vi "Event Log.vi"(11 "Module Config":T1={"Name"="Log", "Parent Q"=refnum, "Is Child?"=FALSE, "Index"=0, "Dirs"={"Root"=path "", "Config"=path "", "Logs"=path "", "Reports"=path "", "App Data"=path ""}, "Simulate"=FALSE, "SimCtrl"=refnum}) -> ()   [LabVIEW 2024, in "EQMF.lvlib" / "Event Log.lvlib"]
uses:
  Event Log.lvlib
  Module/Module Config.ctl
  Queues/Q.Element.ctl
  Module/Module.Working Dirs.ctl
  Module/Module.SW Version Info.ctl
  Module/Window/Window.Task, Action.ctl
  Event Log.Error Report.ctl
  Queues/Queue Utils.lvlib
  Module/Module Utils.lvlib
  Files/File Utils.lvlib
  Controls/Controls.lvlib
panel:
  in  "Main Tab":enum32{"Operate", "Maint"}(tab)
  in  "Clear Errors":bool
  out "Error Count":i32
  out "Log File":path
  in  "Auto Scroll":bool
  out "Event Log":string
  in  "Open Log Folder":bool
  in  "Clear":bool
  in  "Show Block Diagram":bool
  in  "Leave Maint":bool
  in  "Maint":bool
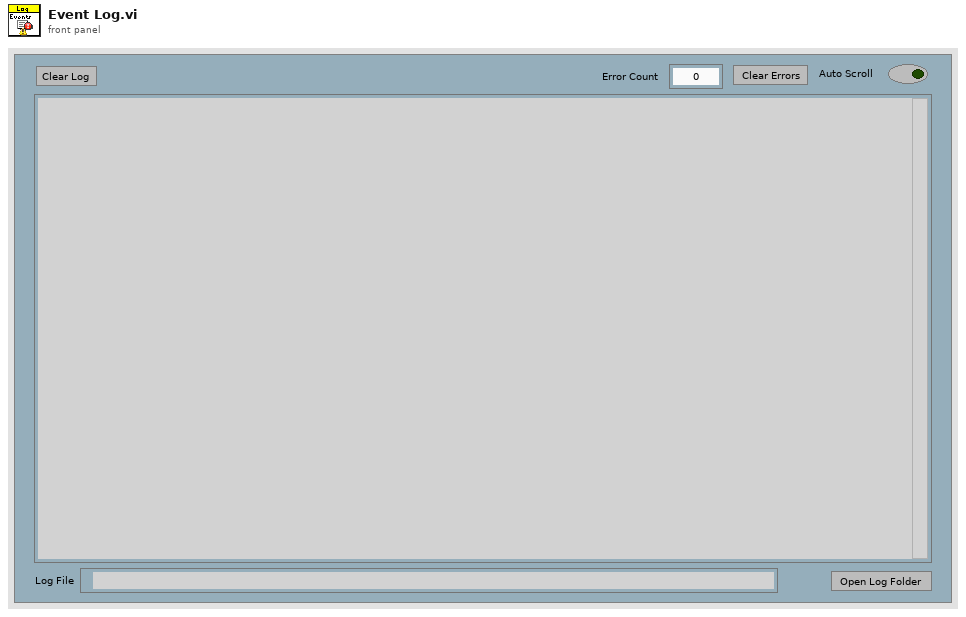
[diagram p1: front panel]
types:
  T1 = typedef "EQMF.lvlib/Module Utils.lvlib/Module Config.ctl" = cluster{"Name":string, "Parent Q":refnum<queue>, "Is Child?":bool, "Index":i32, "Dirs":T2, "Simulate":bool, "SimCtrl":refnum<vi>}
  T2 = typedef "EQMF.lvlib/Module Utils.lvlib/Module.Working Dirs.ctl" = cluster{"Root":path, "Config":path, "Logs":path, "Reports":path, "App Data":path}
  T3 = typedef "EQMF.lvlib/Module Utils.lvlib/Module.SW Version Info.ctl" = cluster{"AppName":string, "Company":string, "Version":string, "Description":string, "PN":string}
  T4 = typedef "EQMF.lvlib/Module Utils.lvlib/Module Sys Info.ctl" = cluster{"Main Q":refnum<queue>, "Exe":bool, "SW Rev":T3, "Self Ref":refnum<vi>, "Main Tab":refnum<vi>, "Pane":refnum<vi>, "Stop":cluster{"Ref":refnum<event-registration>, "Event":refnum<user-event>}, "Cfg":T1, "Services":cluster{"Name":string, "vi ref":refnum<vi>}[], "Menu Ref":refnum<k9>, "CtrlStates":refnum<class "Class.SaveCtrls.lvclass">, "Docs":cluster{"Tags":string[], "Paths":path[]}, "Log":refnum<class "Event Notification.lvclass">, "Test Controls":refnum<vi>[], "Child Modules":cluster{"Name":string, "vi ref":refnum<vi>}[], "SW Items":string[][], "AppData":refnum<class "Class.AppData.lvclass">, "Subscriptions":refnum<class "Subscription.lvclass">, "Module Config Ref":refnum<vi>}
  T5 = typedef "EQMF.lvlib/Module Utils.lvlib/Window.Task, Action.ctl" = enum16{"Resize()", "Show Panel(Bool)", "Show Scroll Bars(Bool)", "Dock to SubPanel(SubPanel Ref)", "Undock from SubPanel()", "Return to SubPanel()", "Go To Maint Tab()", "Show Maint Tab(Bool)", "Open Block Diagram()"}
  T6 = enum16{"Top Left", "Top Right", "Bottom Left", "Bottom Right"}
  T7 = enum16{"Top Left", "Top Right", "Bottom Left", "Bottom Right", "Left", "Right", "Top", "Bottom"}
  T8 = enum16{"open", "replace", "create", "open or create", "replace or create", "replace or create with confirmation"}
  T9 = cluster{"Log":string, "File Ref":refnum<file>, "File Date":string, "Parent Name":string}
  T10 = typedef "EQMF.lvlib/Event Log.lvlib/Event Log.Error Report.ctl" = cluster{"Cnt":i32, "Recent Error":errorcluster}
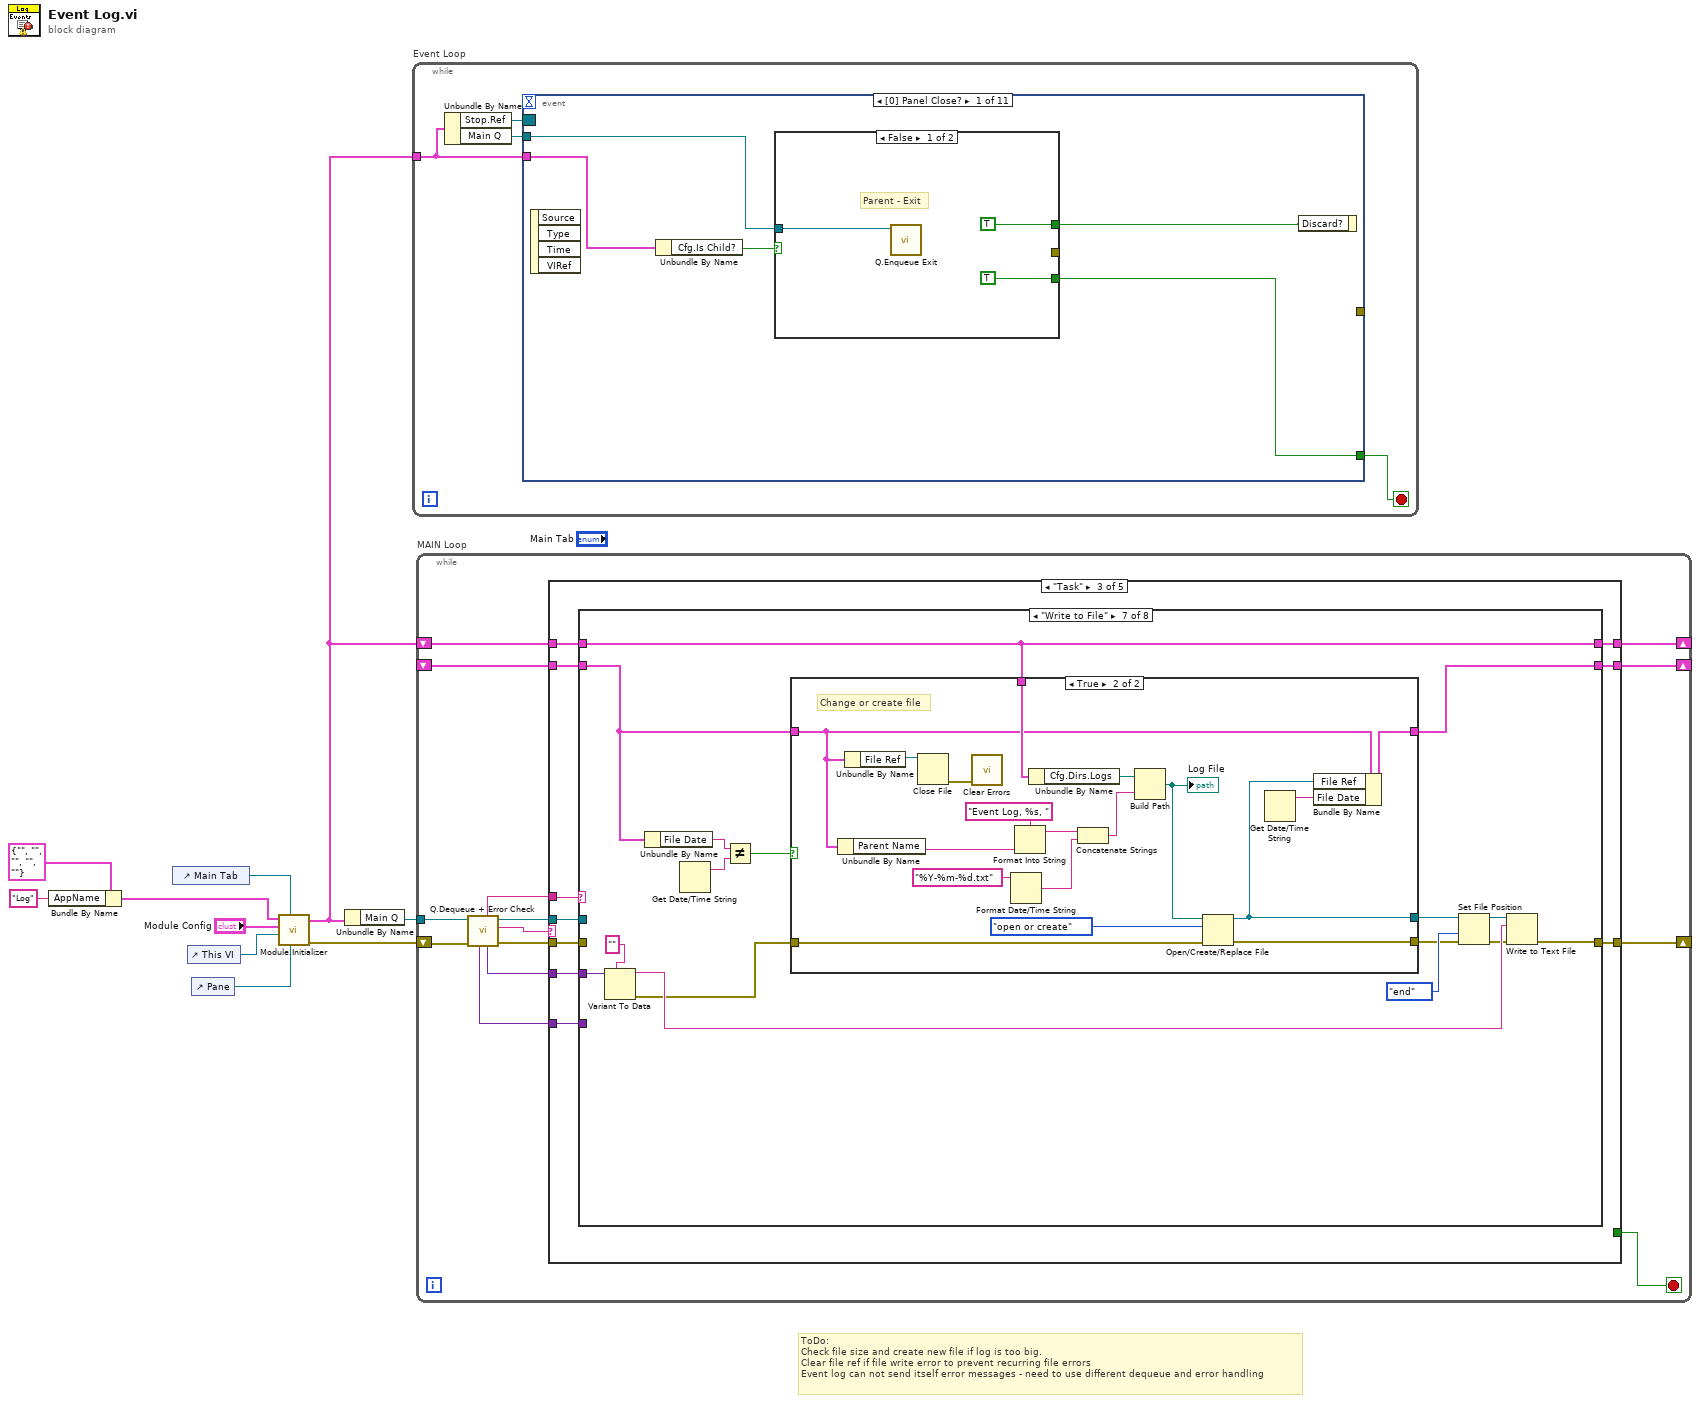
[diagram p0: block diagram]
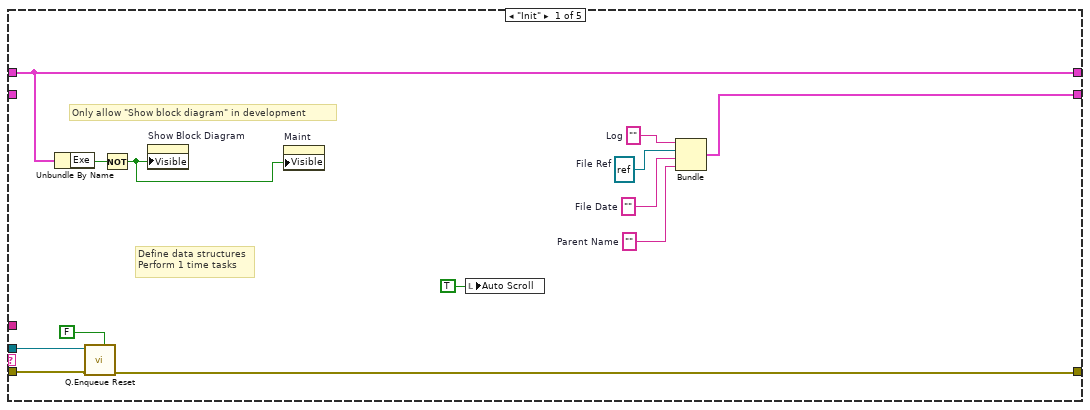
[diagram p2: hidden frame]
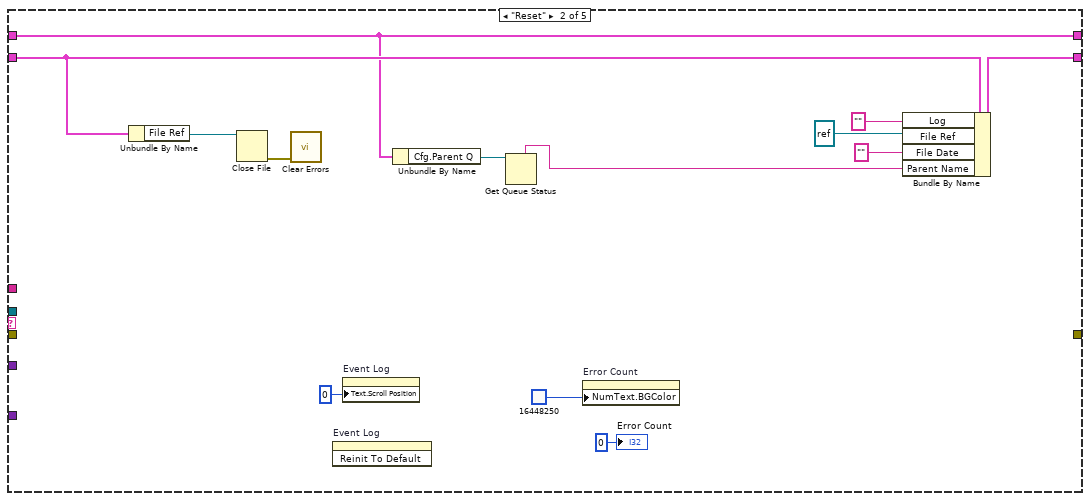
[diagram p3: hidden frame]
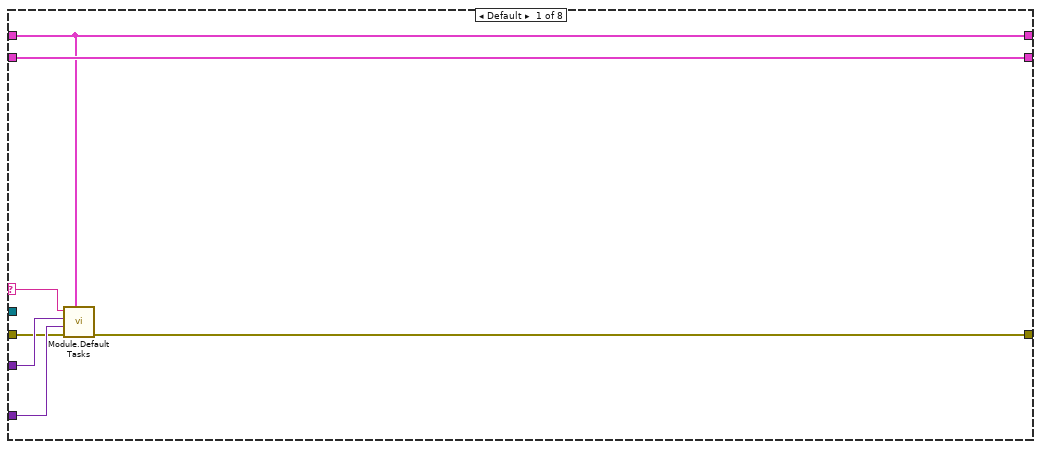
[diagram p4: hidden frame]
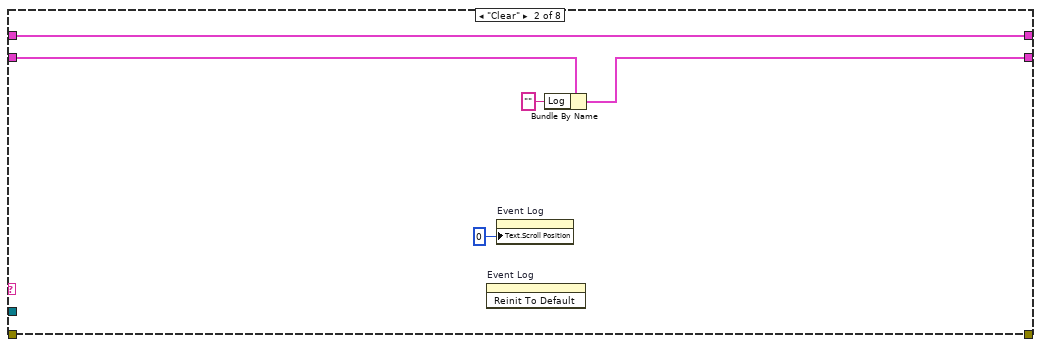
[diagram p5: hidden frame]
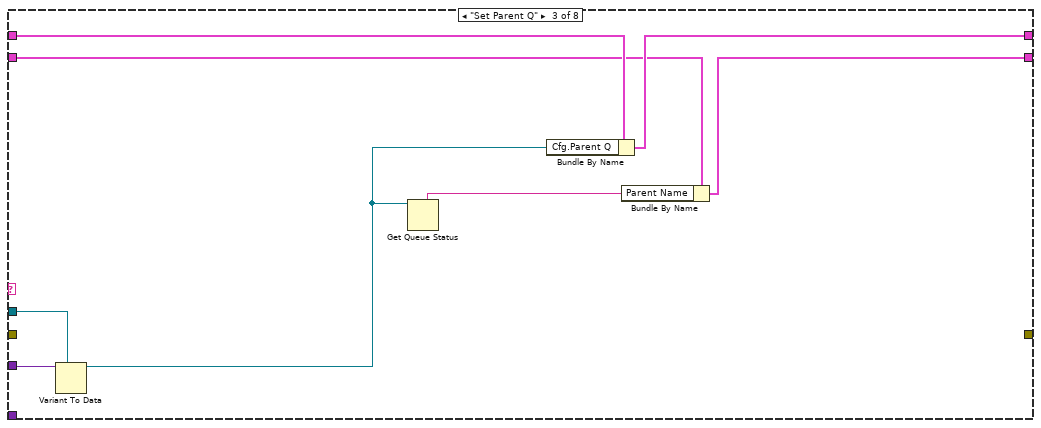
[diagram p6: hidden frame]
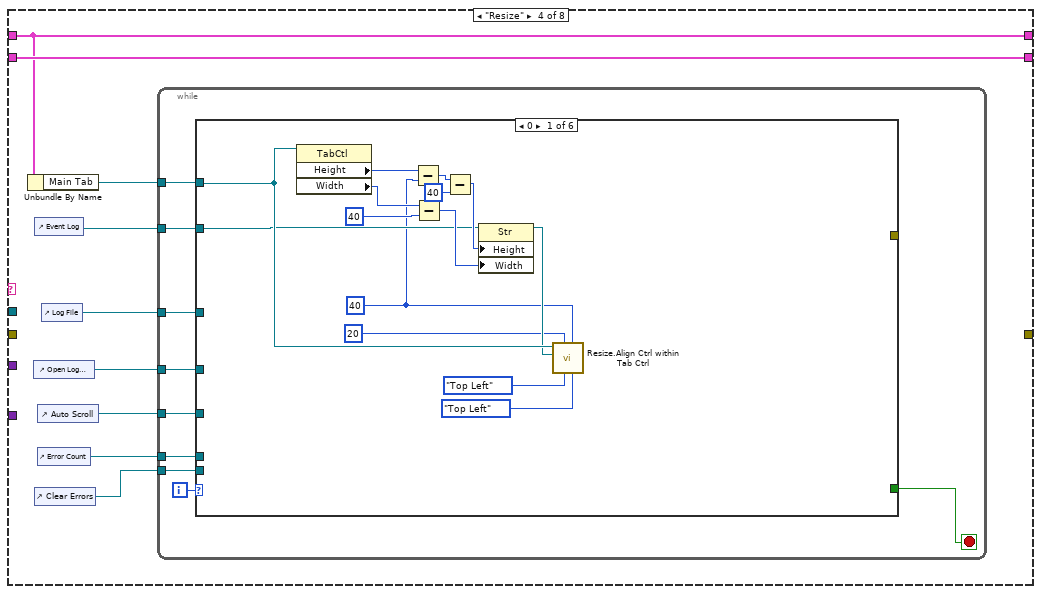
[diagram p7: hidden frame]
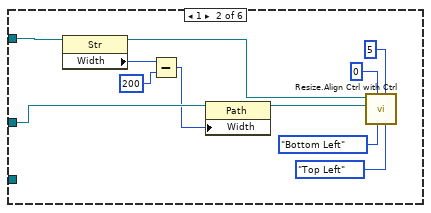
[diagram p8: hidden frame]
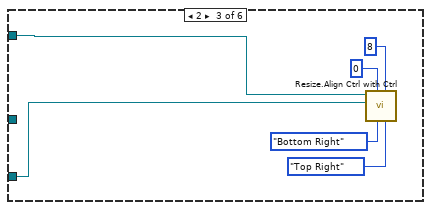
[diagram p9: hidden frame]
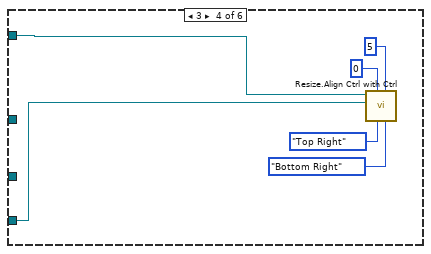
[diagram p10: hidden frame]
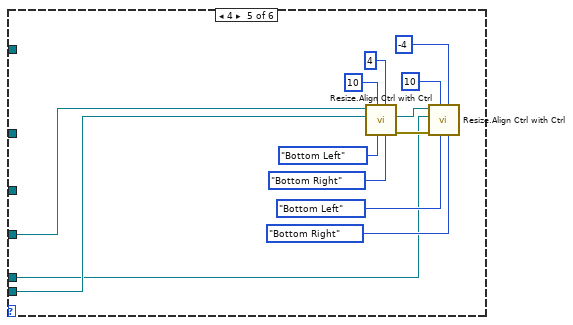
[diagram p11: hidden frame]
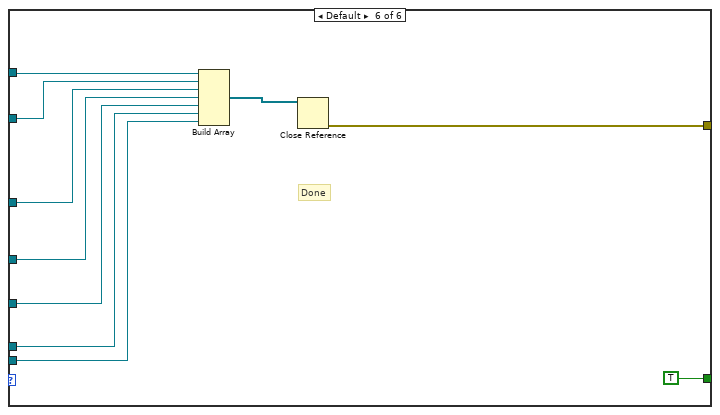
[diagram p12: hidden frame]
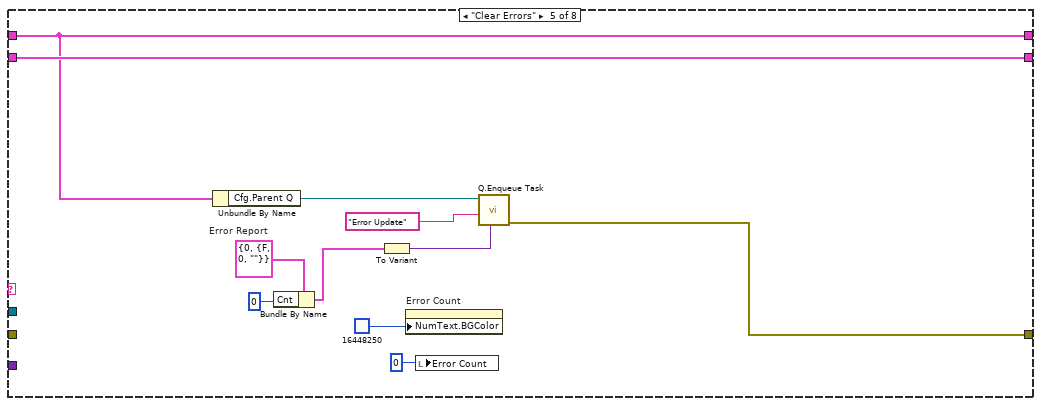
[diagram p13: hidden frame]
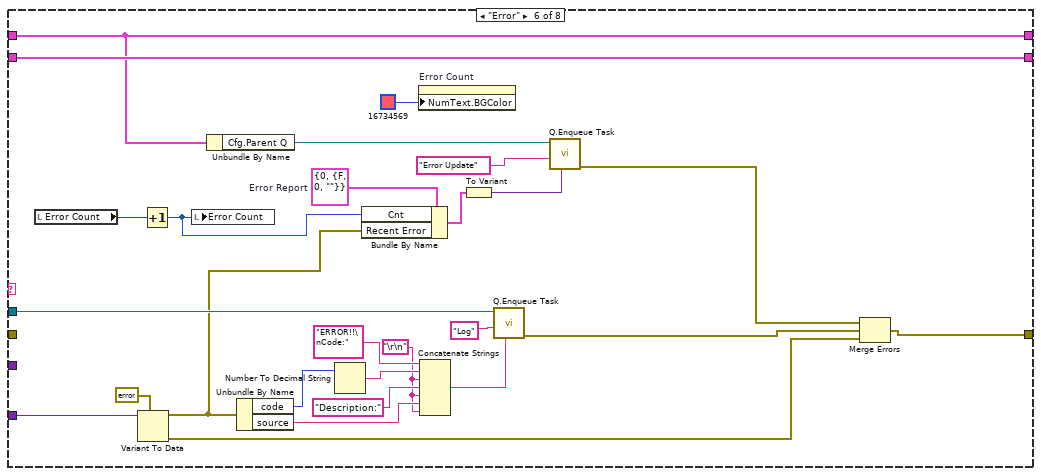
[diagram p14: hidden frame]
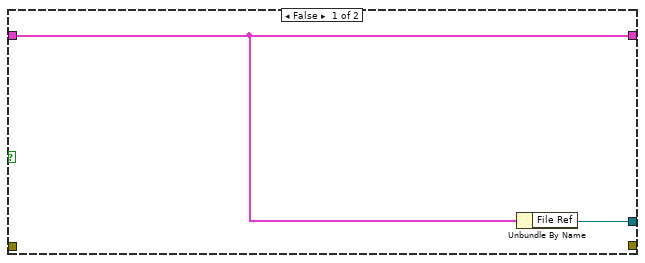
[diagram p15: hidden frame]
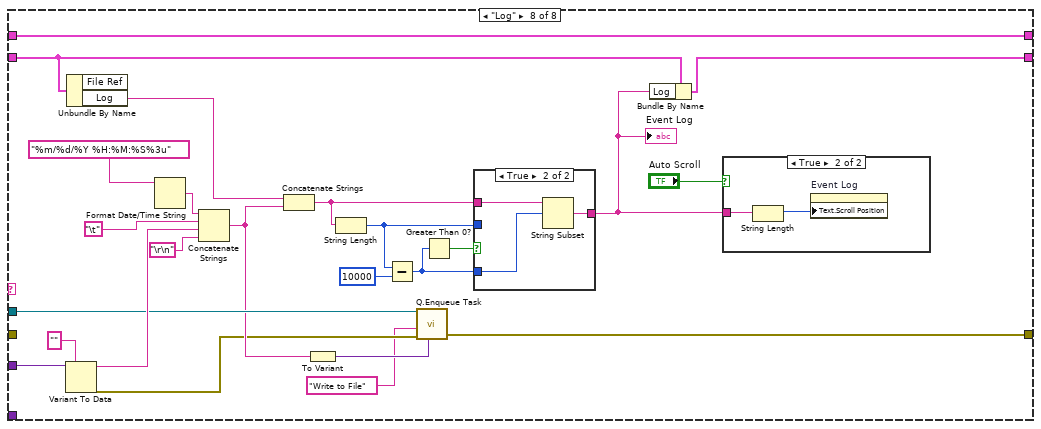
[diagram p16: hidden frame]
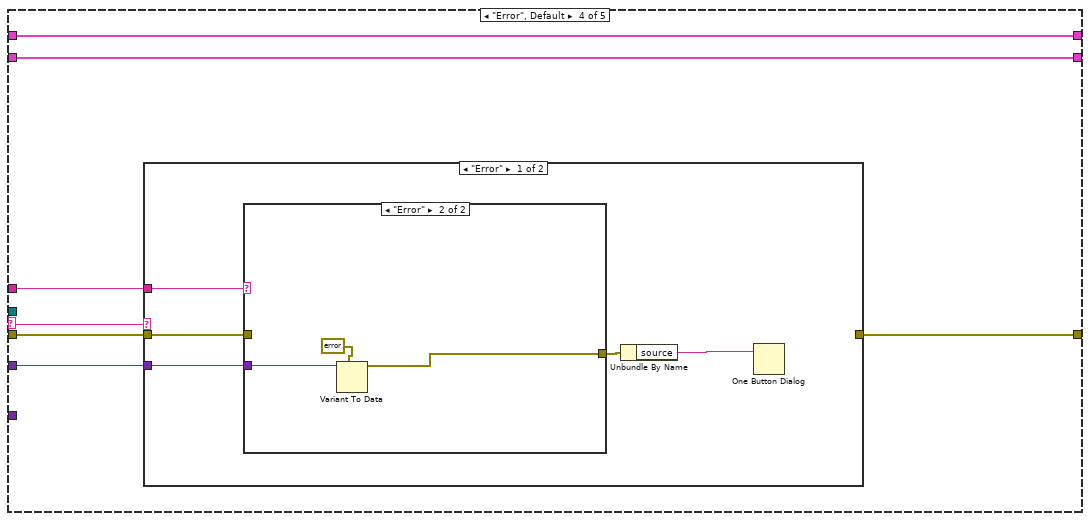
[diagram p19: hidden frame]
diagram:
  # "ToDo:\nCheck file size and create new file if log is too big.\nClear file ref if file write error to prevent recurring file errors \nEvent log can not send itself error messages - need to use different dequeue and error handling"
  n1 = Bundle By Name(cluster=T3 {"AppName"="", "Company"="", "Version"="", "Description"="", "PN"=""} ("SW Rev"), "AppName"="Log") -> (w2:T3)
  n2 = control-ref of="Main Tab"() -> (w6:refnum<vi>)
  n3 = control-ref of="This VI"() -> (w5:refnum<vi>)
  n4 = control-ref of="Pane"() -> (w4:refnum<vi>)
  n5 = call "Module.Initializer.vi"("Pane"=w4, "Main Tab"=w6, "Self Ref"=w5, "Module Config"="Module Config", "SW Rev"=w2) -> ("error out"=w9:errorcluster, "Sys"=w8:T4)  [unwired: 5 in]
  n6 = Unbundle By Name(w8) -> ("Main Q"=w7:refnum<queue>)
  n7 = while "Event Loop" {
    tunnel: w8 -> [w13]
    stop <- w14 stop-if-true
    n8 = Unbundle By Name(w13) -> ("Stop.Ref"=w12:refnum<event-registration>, "Main Q"=w11:refnum<queue>)
    n9 = event shown="[0] Panel Close?" {
      selector: w12 -> [_ _ _ _ _ _ _ _ _ _ _]
      dyn-events: _ -> [_ _ _ _ _ _ _ _ _ _ _]
      timeout: _ -> [_ _ _ _ _ _ _ _ _ _ _]
      tunnel: [w17 _ _ _ _ _ _ _ _ w46 TRUE] -> w14
      tunnel: w13 -> [w16 _ _ _ _ w37 _ _ _ _ _]
      tunnel: w11 -> [w19 w29 w31 w33 w35 _ _ w43 _ w45 _]
      tunnel: [_ _ _ _ _ w38 _ _ _ _ _] -> _
      event Panel Close? {
        n10 = event-data() -> ()  [unwired: 1 in, 4 out]
        n11 = Unbundle By Name(w16) -> ("Cfg.Is Child?"=w15:bool)
        n12 = case shown="False" w15 {
          tunnel: w19 -> [w22 w25]
          tunnel: [TRUE TRUE] -> w18
          tunnel: [TRUE FALSE] -> w17
          tunnel: [_ w23] -> _
          frame False {
            # "Parent - Exit"
            n13 = call "Q.Enqueue Exit.vi"("Q In"=w22) -> ()  [unwired: 9 in, 2 out]
          }
          frame True {
            # "Child - Hide Panel"
            n14 = call "Module.Window, Q Task.vi"("Action"=Window.Task,_Action."Show Panel(Bool)", "Q In"=w25) -> ("error out"=w23:errorcluster)  [unwired: 8 in, 1 out]
          }
        }
        n15 = event-data("Discard?"=w18) -> ()  [unwired: 1 in, 1 out]
      }
      event Panel Resize {
        n16 = event-data() -> ()  [unwired: 1 in, 8 out]
        n17 = call "Module.Window, Q Task.vi"("Action"=Window.Task,_Action."Resize()", "Q In"=w29) -> ()  [unwired: 8 in, 2 out]
      }
      event "Show Block Diagram": Value Change {
        n18 = event-data() -> ()  [unwired: 1 in, 6 out]
        n19 = call "Module.Window, Q Task.vi"("Action"=Window.Task,_Action."Open Block Diagram()", "Q In"=w31) -> ()  [unwired: 8 in, 2 out]
      }
      event "Maint": Value Change {
        n20 = event-data() -> ()  [unwired: 1 in, 6 out]
        n21 = call "Module.Window, Q Task.vi"("Action"=Window.Task,_Action."Go To Maint Tab()", "Q In"=w33) -> ()  [unwired: 8 in, 2 out]
      }
      event "Clear Errors": Value Change {
        n22 = event-data() -> ()  [unwired: 1 in, 6 out]
        n23 = call "Q.Enqueue Task.vi"("Task Name"="Clear Errors", "Q In"=w35) -> ()  [unwired: 8 in, 2 out]
      }
      event "Open Log Folder": Value Change {
        n24 = event-data() -> ()  [unwired: 1 in, 6 out]
        n25 = Unbundle By Name(w37) -> ("Cfg.Dirs.Logs"=w36:path)
        n26 = call "File.Open File or Folder.vi"("Path"=w36) -> ("Error Out"=w38:errorcluster)  [unwired: 10 in]
      }
      event "Auto Scroll": Value Change {
        n27 = event-data() -> ("NewVal"=w39:bool)  [unwired: 1 in, 5 out]
        n28 = case shown="True" w39 {
          frame False {
          }
          frame True {
            n29 = local read "Event Log"() -> (w41:string)
            n30 = String Length(string=w41) -> (length=w40:i32)
            n31 = property on="Event Log" class="Str"("Text.Scroll Position"=w40) -> ()  [unwired: 2 in, 2 out]
          }
        }
      }
      event "Clear": Value Change {
        n32 = event-data() -> ()  [unwired: 1 in, 6 out]
        n33 = call "Q.Enqueue Task.vi"("Task Name"="Clear", "Q In"=w43) -> ()  [unwired: 8 in, 2 out]
      }
      event "Leave Maint": Value Change {
        n34 = event-data() -> ()  [unwired: 1 in, 6 out]
        n35 = local write "Main Tab"(0) -> ()
      }
      event Menu Selection (User) {
        n36 = event-data() -> ("ItemTag"=w47:string)  [unwired: 1 in, 6 out]
        n37 = case shown="\"Exit\"" w47 {
          tunnel: [_ TRUE] -> w46
          tunnel: w45 -> [_ w48]
          frame "False", Default {
          }
          frame "Exit" {
            n38 = call "Q.Enqueue Exit.vi"("Q In"=w48) -> ()  [unwired: 9 in, 2 out]
          }
        }
      }
      event User Event {
        n39 = event-data() -> ()  [unwired: 1 in, 5 out]
      }
    }
  }
  n40 = while "MAIN Loop" {
    shift-right: [w60] -> _
    shift-left: w9 -> [w58]
    shift-right: [w61] -> _
    shift-left: _ -> [w64]
    shift-right: [w62] -> _
    shift-left: w8 -> [w63]
    tunnel: w7 -> [w57]
    stop <- w51 stop-if-true
    n41 = call "Q.Dequeue + Error Check.vi"("Error In"=w58, "Q In"=w57) -> ("error out"=w59:errorcluster, "Cmd"=w56:string, "Q Out"=w55:refnum<queue>, "Data1"=w54:variant, "Sub"=w52:string, "Data2"=w53:variant)  [unwired: 4 in]
    n42 = case shown="\"Task\"" w56 {
      selector: w56 -> [_ _ _ w305 _]
      tunnel: w64 -> [_ w81 w99 w307 w333]
      tunnel: w63 -> [w71 w80 w100 w308 w335]
      tunnel: [w71 w80 w98 w308 w335] -> w62
      tunnel: [w72 w90 w97 w307 w333] -> w61
      tunnel: [w74 _ w91 w306 w337] -> w60
      tunnel: w59 -> [w75 _ w93 w303 w336]
      tunnel: w55 -> [w76 _ w94 _ _]
      tunnel: w54 -> [_ _ w95 w304 _]
      tunnel: w53 -> [_ _ w92 _ _]
      tunnel: w52 -> [_ _ w96 w302 _]
      tunnel: [_ _ _ _ TRUE] -> w51
      frame "Init" {
        w65 = ""  # Parent Name
        w68 = ""  # File Date
        w69 = refnum<file> refnum  # File Ref
        w77 = ""  # Log
        # "Only allow \"Show block diagram\" in development"
        # "Define data structures\nPerform 1 time tasks"
        n43 = Unbundle By Name(w71) -> ("Exe"=w70:bool)
        n44 = call "Q.Enqueue Reset.vi"("Top of Q(T)"=FALSE ("Flush Q"), "Error In"=w75, "Q In"=w76) -> ("error out"=w74:errorcluster)  [unwired: 7 in, 1 out]
        n45 = Not(x=w70) -> (.not. x?=w67:bool)
        n46 = property on="Show Block Diagram" class="Bool"("Visible"=w67) -> ()  [unwired: 2 in, 2 out]
        n47 = property on="Maint" class="Bool"("Visible"=w67) -> ()  [unwired: 2 in, 2 out]
        n48 = local write "Auto Scroll"(TRUE ("Auto Scroll")) -> ()
        n49 = Bundle("Log"=w77, "File Ref"=w69, "File Date"=w68, "Parent Name"=w65) -> (w72:T9)  [unwired: 1 in]
      }
      frame "Reset" {
        n50 = Unbundle By Name(w81) -> ("File Ref"=w89:refnum<file>)
        n51 = Close File(refnum=w89) -> (error out=w88:errorcluster)  [unwired: 1 in, 1 out]
        n52 = call <vilib>:"Clear Errors.vi"("error in (no error)"=w88) -> ()  [unwired: 5 in, 2 out]
        n53 = invoke on="Event Log" class="Str" method="Reinit To Default"() -> ()  [unwired: 3 in, 3 out]
        n54 = property on="Event Log" class="Str"("Text.Scroll Position"=u32 0) -> ()  [unwired: 2 in, 2 out]
        n55 = Unbundle By Name(w80) -> ("Cfg.Parent Q"=w79:refnum<queue>)
        n56 = Get Queue Status(queue=w79) -> (queue name=w78:string)  [unwired: 2 in, 7 out]
        n57 = property on="Error Count" class="DigNum (strict)"("NumText.BGColor"=u32 16448250) -> ()  [unwired: 2 in, 2 out]
        n58 = Bundle By Name(cluster=w81, "Log"="", "File Ref"=refnum<file> refnum, "File Date"="", "Parent Name"=w78) -> (w90:T9)
        "Error Count" <- 0 ("Error Count")
      }
      frame "Task" {
        n59 = case shown="\"Write to File\"" w96 {
          selector: w96 -> [w105 _ _ _ _ _ _ _]
          tunnel: w100 -> [w106 w112 w118 w128 w207 w223 w250 w295]
          tunnel: w99 -> [w107 w111 w115 w129 w209 w235 w249 w280]
          tunnel: [w106 w112 w117 w128 w207 w223 w250 w295] -> w98
          tunnel: [w107 w110 w114 w129 w209 w235 w251 w279] -> w97
          tunnel: w95 -> [w104 _ w120 _ _ _ w246 w281]
          tunnel: w94 -> [_ _ w119 _ _ w222 _ w278]
          tunnel: w93 -> [w102 _ _ _ _ _ _ _]
          tunnel: w92 -> [w103 _ _ _ _ w221 _ _]
          tunnel: [w101 _ _ _ w204 w219 w244 w274] -> w91
          frame Default {
            n60 = call "Module.Default Tasks.vi"("Sys"=w106, "error in"=w102, "Data2"=w103, "Data1"=w104, "Sub"=w105) -> ("error out"=w101:errorcluster)  [unwired: 5 in, 1 out]
          }
          frame "Clear" {
            n61 = invoke on="Event Log" class="Str" method="Reinit To Default"() -> ()  [unwired: 3 in, 3 out]
            n62 = property on="Event Log" class="Str"("Text.Scroll Position"=u32 0) -> ()  [unwired: 2 in, 2 out]
            n63 = Bundle By Name(cluster=w111, "Log"="") -> (w110:T9)
          }
          frame "Set Parent Q" {
            n64 = Variant To Data(type=w119, Variant=w120) -> (data=w116:refnum<queue>)  [unwired: 1 in, 1 out]
            n65 = Get Queue Status(queue=w116) -> (queue name=w113:string)  [unwired: 2 in, 7 out]
            n66 = Bundle By Name(cluster=w118, "Cfg.Parent Q"=w116) -> (w117:T4)
            n67 = Bundle By Name(cluster=w115, "Parent Name"=w113) -> (w114:T9)
          }
          frame "Resize" {
            n68 = Unbundle By Name(w128) -> ("Main Tab"=w127:refnum<vi>)
            n69 = control-ref of="Open Log Folder"() -> (w124:refnum<vi>)
            n70 = control-ref of="Event Log"() -> (w126:refnum<vi>)
            n71 = control-ref of="Clear Errors"() -> (w121:refnum<vi>)
            n72 = control-ref of="Auto Scroll"() -> (w123:refnum<vi>)
            n73 = control-ref of="Error Count"() -> (w122:refnum<vi>)
            n74 = control-ref of="Log File"() -> (w125:refnum<vi>)
            n75 = while {
              tunnel: w127 -> [w136]
              tunnel: w126 -> [w135]
              tunnel: w125 -> [w134]
              tunnel: w124 -> [w133]
              tunnel: w123 -> [w132]
              tunnel: w122 -> [w131]
              tunnel: w121 -> [w130]
              i -> [w138]
              stop <- w137 stop-if-true
              n76 = case shown="0" w138 {
                tunnel: [_ _ _ _ _ TRUE] -> w137
                tunnel: w136 -> [w150 _ _ _ _ w197]
                tunnel: w135 -> [w141 w159 w165 w171 _ w196]
                tunnel: w134 -> [_ w158 _ _ _ w195]
                tunnel: w133 -> [_ _ w164 _ _ w194]
                tunnel: w132 -> [_ _ _ w170 w185 w193]
                tunnel: w131 -> [_ _ _ _ w176 w192]
                tunnel: w130 -> [_ _ _ _ w177 w191]
                tunnel: [_ _ _ _ _ w189] -> _
                frame 0 {
                  w140 = u32 40 ("y")
                  n77 = property class="TabCtl"(reference=w150) -> ("Height"=w149:u32, "Width"=w148:u32)  [unwired: 1 in, 2 out]
                  n78 = Subtract(x=w149, y=w140) -> (x-y=w145:u32)
                  n79 = Subtract(x=w148, y=u32 40) -> (x-y=w146:u32)
                  n80 = Subtract(x=w145, y=u32 40) -> (x-y=w143:u32)
                  n81 = property class="Str"(reference=w141, "Height"=w143, "Width"=w146) -> (reference out=w142:refnum<vi>)  [unwired: 1 in, 1 out]
                  n82 = call "Resize.Align Ctrl within Tab Ctrl.vi"("Child Ref Pos"=T6."Top Left", "dY"=w140, "Parent Ref Pos"=T6."Top Left", "dX"=u32 20 ("y"), "Child Ctrl"=w142, "Parent Tab Ctrl"=w150) -> ()  [unwired: 3 in, 3 out]
                }
                frame 1 {
                  n83 = property class="Str"(reference=w159) -> (reference out=w156:refnum<vi>, "Width"=w157:u32)  [unwired: 1 in, 1 out]
                  n84 = Subtract(x=w157, y=200) -> (x-y=w154:u32)
                  n85 = property class="Path"(reference=w158, "Width"=w154) -> (reference out=w153:refnum<vi>)  [unwired: 1 in, 1 out]
                  n86 = call "Resize.Align Ctrl with Ctrl.vi"("Move Ctrl Ref Location"=T7."Top Left", "dY"=5, "Ref Ctrl Corner"=T6."Bottom Left", "dX"=0, "Move Ctrl"=w153, "Ref Ctrl"=w156) -> ()  [unwired: 3 in, 3 out]
                }
                frame 2 {
                  n87 = call "Resize.Align Ctrl with Ctrl.vi"("Move Ctrl Ref Location"=T7."Top Right", "dY"=8, "Ref Ctrl Corner"=T6."Bottom Right", "dX"=0, "Move Ctrl"=w164, "Ref Ctrl"=w165) -> ()  [unwired: 3 in, 3 out]
                }
                frame 3 {
                  n88 = call "Resize.Align Ctrl with Ctrl.vi"("Move Ctrl Ref Location"=T7."Bottom Right", "dY"=5, "Ref Ctrl Corner"=T6."Top Right", "dX"=0, "Move Ctrl"=w170, "Ref Ctrl"=w171) -> ()  [unwired: 3 in, 3 out]
                }
                frame 4 {
                  n89 = call "Resize.Align Ctrl with Ctrl.vi"("Move Ctrl Ref Location"=T7."Bottom Right", "dY"=4, "Ref Ctrl Corner"=T6."Bottom Left", "dX"=10, "Move Ctrl"=w177, "Ref Ctrl"=w185) -> ("error out"=w184:errorcluster, "Move Ctrl Out"=w181:refnum<vi>)  [unwired: 3 in, 1 out]
                  n90 = call "Resize.Align Ctrl with Ctrl.vi"("Move Ctrl Ref Location"=T7."Bottom Right", "dY"=-4, "Ref Ctrl Corner"=T6."Bottom Left", "dX"=10 ("dY"), "error in"=w184, "Move Ctrl"=w176, "Ref Ctrl"=w181) -> ()  [unwired: 2 in, 3 out]
                }
                frame Default {
                  # "Done"
                  n91 = Build Array(w197, w196, w195, w194, w193, w192, w191) -> (w190:refnum<vi>[])
                  n92 = Close Reference(reference=w190) -> (error out=w189:errorcluster)  [unwired: 1 in]
                }
              }
            }
          }
          frame "Clear Errors" {
            w203 = T10 {"Cnt"=0, "Recent Error"={"status"=FALSE, "code"=0, "source"=""}}  # Error Report
            n93 = Unbundle By Name(w207) -> ("Cfg.Parent Q"=w208:refnum<queue>)
            n94 = Bundle By Name(cluster=w203, "Cnt"=0) -> (w201:T10)
            n95 = To Variant(anything=w201) -> (Variant=w200:variant)
            n96 = property on="Error Count" class="DigNum (strict)"("NumText.BGColor"=u32 16448250) -> ()  [unwired: 2 in, 2 out]
            n97 = local write "Error Count"(0 ("Error Count")) -> ()
            n98 = call "Q.Enqueue Task.vi"("Data1"=w200, "Task Name"="Error Update", "Q In"=w208) -> ("error out"=w204:errorcluster)  [unwired: 7 in, 1 out]
          }
          frame "Error" {
            w217 = T10 {"Cnt"=0, "Recent Error"={"status"=FALSE, "code"=0, "source"=""}}  # Error Report
            w218 = "\r\n"
            n99 = local read "Error Count"() -> (w234:i32)
            n100 = Variant To Data(type=errorcluster {"status"=FALSE, "code"=0, "source"=""} ("error constant"), Variant=w221) -> (data=w214:errorcluster, error out=w224:errorcluster)  [unwired: 1 in]
            n101 = Increment(x=w234) -> (x+1=w215:i32)
            n102 = local write "Error Count"(w215) -> ()
            n103 = Unbundle By Name(w223) -> ("Cfg.Parent Q"=w232:refnum<queue>)
            n104 = Unbundle By Name(w214) -> ("code"=w227:i32, "source"=w229:string)
            n105 = Number To Decimal String(number=w227) -> (decimal integer string=w226:string)  [unwired: 1 in]
            n106 = Bundle By Name(cluster=w217, "Cnt"=w215, "Recent Error"=w214) -> (w216:T10)
            n107 = property on="Error Count" class="DigNum (strict)"("NumText.BGColor"=u32 16734569) -> ()  [unwired: 2 in, 2 out]
            n108 = Concatenate Strings("ERROR!!\nCode:", w226, w218, "Description:", w218, w229, w218) -> (w211:string)
            n109 = To Variant(anything=w216) -> (Variant=w213:variant)
            n110 = call "Q.Enqueue Task.vi"("Data1"=w211, "Task Name"="Log", "Q In"=w222) -> ("error out"=w220:errorcluster)  [unwired: 7 in, 1 out]
            n111 = call "Q.Enqueue Task.vi"("Data1"=w213, "Task Name"="Error Update", "Q In"=w232) -> ("error out"=w230:errorcluster)  [unwired: 7 in, 1 out]
            n112 = Merge Errors(w230, w220, w224) -> (w219:errorcluster)
          }
          frame "Write to File" {
            n113 = Variant To Data(type="", Variant=w246) -> (data=w243:string, error out=w242:errorcluster)  [unwired: 1 in]
            n114 = Unbundle By Name(w249) -> ("File Date"=w248:string)
            n115 = Get Date/Time String() -> (date string=w247:string)  [unwired: 3 in, 1 out]
            n116 = Not Equal?(x=w248, y=w247) -> (x != y?=w241:bool)
            n117 = case shown="True" w241 {
              tunnel: [w253 w262] -> w251
              tunnel: w250 -> [_ w261]
              tunnel: w249 -> [w253 w255]
              tunnel: [_ w260] -> w239
              tunnel: [w252 w259] -> w238
              tunnel: w242 -> [_ w258]
              frame False {
                n118 = Unbundle By Name(w253) -> ("File Ref"=w252:refnum<file>)
              }
              frame True {
                # "Change or create file"
                n119 = Unbundle By Name(w255) -> ("Parent Name"=w254:string)
                n120 = Unbundle By Name(w255) -> ("File Ref"=w271:refnum<file>)
                n121 = Close File(refnum=w271) -> (error out=w270:errorcluster)  [unwired: 1 in, 1 out]
                n122 = call <vilib>:"Clear Errors.vi"("error in (no error)"=w270) -> ()  [unwired: 5 in, 2 out]
                n123 = Format Date/Time String(time format string (%c)="%Y-%m-%d.txt") -> (date/time string=w267:string)  [unwired: 2 in]
                n124 = Format Into String(format string="Event Log, %s, ", w254) -> (resulting string=w256:string)  [unwired: 2 in, 1 out]
                n125 = Unbundle By Name(w261) -> ("Cfg.Dirs.Logs"=w268:path)
                n126 = Concatenate Strings(w256, w267) -> (w265:string)
                n127 = Build Path(base path=w268, name or relative path=w265) -> (appended path=w269:path)
                "Log File" <- w269
                n128 = Open/Create/Replace File(file path (use dialog)=w269, error in=w258, operation (0:open)=T8."open or create") -> (refnum out=w259:refnum<file>, error out=w260:errorcluster)  [unwired: 3 in, 1 out]
                n129 = Get Date/Time String() -> (date string=w263:string)  [unwired: 3 in, 1 out]
                n130 = Bundle By Name(cluster=w255, "File Ref"=w259, "File Date"=w263) -> (w262:T9)
              }
            }
            n131 = Set File Position(refnum=w238, from (0:start)=enum16{"start", "end", "current"}."end", error in=w239) -> (refnum out=w237:refnum<file>, error out=w236:errorcluster)  [unwired: 1 in]
            n132 = Write to Text File(file (use dialog)=w237, text=w243, error in=w236) -> (error out=w244:errorcluster)  [unwired: 1 in, 2 out]
          }
          frame "Log" {
            n133 = Variant To Data(type="", Variant=w281) -> (data=w291:string, error out=w275:errorcluster)  [unwired: 1 in]
            n134 = Unbundle By Name(w280) -> ("Log"=w282:string)  [unwired: 1 out]
            n135 = Format Date/Time String(time format string (%c)="%m/%d/%Y %H:%M:%S%3u") -> (date/time string=w293:string)  [unwired: 2 in]
            n136 = Concatenate Strings(w293, "\t", w291, "\r\n") -> (w276:string)
            n137 = Concatenate Strings(w282, w276) -> (w285:string)
            n138 = To Variant(anything=w276) -> (Variant=w277:variant)
            n139 = String Length(string=w285) -> (length=w287:i32)
            n140 = Subtract(x=w287, y=10000) -> (x-y=w286:i32)
            n141 = call "Q.Enqueue Task.vi"("Data1"=w277, "Error In"=w275, "Task Name"="Write to File", "Q In"=w278) -> ("error out"=w274:errorcluster)  [unwired: 6 in, 1 out]
            n142 = Greater Than 0?(x=w286) -> (x > 0?=w288:bool)
            n143 = case shown="True" w288 {
              tunnel: w287 -> [_ _]
              tunnel: w286 -> [_ w300]
              tunnel: w285 -> [w298 w301]
              tunnel: [w298 w299] -> w283
              frame False {
              }
              frame True {
                n144 = String Subset(string=w301, offset (0)=w300) -> (substring=w299:string)  [unwired: 1 in]
              }
            }
            "Event Log" <- w283
            n145 = Bundle By Name(cluster=w280, "Log"=w283) -> (w279:T9)
            n146 = case shown="True" "Auto Scroll" {
              tunnel: w283 -> [_ w297]
              frame False {
              }
              frame True {
                n147 = String Length(string=w297) -> (length=w296:i32)
                n148 = property on="Event Log" class="Str"("Text.Scroll Position"=w296) -> ()  [unwired: 2 in, 2 out]
              }
            }
          }
        }
      }
      frame "Error", Default {
        n149 = case shown="\"Error\"" w305 {
          selector: w305 -> [_ w318]
          tunnel: [_ w319] -> w306
          tunnel: w304 -> [w313 _]
          tunnel: w303 -> [w309 _]
          tunnel: w302 -> [w312 _]
          frame "Error" {
            n150 = case shown="\"Error\"" w312 {
              tunnel: w313 -> [_ w317]
              tunnel: [w314 w315] -> w310
              tunnel: w309 -> [w314 _]
              frame "", Default {
              }
              frame "Error" {
                n151 = Variant To Data(type=errorcluster {"status"=FALSE, "code"=0, "source"=""} ("error constant"), Variant=w317) -> (data=w315:errorcluster)  [unwired: 1 in, 1 out]
              }
            }
            n152 = Unbundle By Name(w310) -> ("source"=w311:string)
            n153 = One Button Dialog(message=w311) -> ()  [unwired: 1 in, 1 out]
          }
          frame Default {
            n154 = Concatenate Strings("Undefined State: \"", w318, "\".") -> (w320:string)
            n155 = Bundle By Name(cluster=errorcluster {"status"=TRUE, "code"=-5000, "source"=""} ("error constant"), "source"=w320) -> (w319:errorcluster)
          }
        }
      }
      frame "Exit" {
        n156 = Unbundle By Name(w333) -> ("File Ref"=w326:refnum<file>)
        n157 = Format Date/Time String() -> (date/time string=w329:string)  [unwired: 3 in]
        n158 = Concatenate Strings(w329, "\t", "Application Exit", "\r\n") -> (w331:string)
        n159 = Write to Text File(file (use dialog)=w326, text=w331) -> (refnum out=w324:refnum<file>, error out=w325:errorcluster)  [unwired: 2 in, 1 out]
        n160 = Close File(refnum=w324, error in=w325) -> (error out=w332:errorcluster)  [unwired: 1 out]
        n161 = call <vilib>:"Clear Errors.vi"("error in (no error)"=w332) -> ()  [unwired: 5 in, 2 out]
        n162 = call "Module.Destructor.vi"("error in"=w336, "Sys"=w335) -> ("error out"=w337:errorcluster)  [unwired: 9 in]
      }
    }
  }
